vi "UHR-Fleezers Control (host) - 11.9b.vi"() -> ()   [LabVIEW 2014] (continued)
                n2360 = call "Create new save file.vi"("Insert"="video_frame_" ("string"), "Ext"=".bmp" ("string"), "Index In"="Image Index") -> ("Path Out"=w3445:path, "Index Out"=w3450:dbl)
                n2361 = Increment(x=w3450) -> (x+1=w3444:dbl)
                n2362 = local write "Image Index"(w3444) -> ()
                n2363 = call <vilib>:"Write BMP File.vi"("image data"=w3449, "path to BMP file"=w3445) -> ()  [unwired: 1 in, 9 out]
              }
            }
            n2364 = case shown="True" "Target" {
              tunnel: w3363 -> [w3389 w3393]
              tunnel: [w3389 w3391] -> w3362
              frame False {
              }
              frame True {
                n2365 = local read "Target coordinates"() -> (w3390:cluster{"X1":dbl, "Y1":dbl, "X2":dbl, "Y2":dbl})
                n2366 = call "IMAQ Overlay Oval"("Color"=u32 16711680, "Bounding Rectangle"=w3390, "Image"=w3393) -> ("Image Out"=w3391:T2)  [unwired: 7 in, 1 out]
              }
            }
            "Primary Video Display" <- w3362
          }
        }
        n2367 = node-c288(w3324) -> ()  [unwired: 1 out]
      }
      n2368 = node-c288(w3308) -> ()  [unwired: 1 out]
      n2369 = call "DMR_CloseDevice2.vi"("driver handle IN"=w3313) -> ()  [unwired: 1 in, 4 out]
    }
    frame #4 {
      n2370 = call "DMR_Close.vi"() -> ()  [unwired: 1 out]
    }
  }
  n2371 = local write "Offset (nm)"(0.0 ("Offset (nm)")) -> ()
  n2372 = local write "Bead Mean (nm)"(0.0 ("Bead Mean (nm)")) -> ()
  n2373 = local write "Total Volume\nFlowed P1 (uL)"(w17) -> ()
  n2374 = local write "Total Volume\nFlowed Samp (uL)"(w17) -> ()
  n2375 = local write "Total Volume\nFlowed P3 (uL)"(w17) -> ()
  n2376 = node-c288(i64 1 ("Period"), 1 ("Processor")) -> (w196:T21)  [unwired: 2 out]
  n2377 = timed-loop "Acquire Data" {
    tunnel: w23 -> [w3758]
    tunnel: w72 -> [w3757]
    tunnel: [w3787] -> w289
    tunnel: [w3782] -> w287
    timing: w196 -> [_]
    timing-out: [_] -> w195
    tunnel: w91 -> [w3597]
    stop <- "Stop All" stop-if-true
    w3515 = "Initialize"
    w3584 = "NI_ChannelName" ("name")
    # "I think that the conversion\nfrom 'wiggle amp' to nm\nis 0.277 nm/input. So, 1000\nfor an input is 277 nm."
    n2378 = node-c288() -> ()  [unwired: 2 out]
    n2379 = First Call?() -> (First Call?: T/F=w3550:bool)
    n2380 = Or(x="Reset", y=w3550) -> (x .or. y?=w3551:bool)
    n2381 = local read "Flushing P1"() -> (w3470:bool)
    n2382 = case "Reset data stream" shown="True" w3551 {
      tunnel: w3758 -> [w4825 w4833]
      tunnel: w3757 -> [w4824 w4832]
      tunnel: [w4825 w4827] -> w3463
      tunnel: [w4824 w4826] -> w3753
      frame False {
      }
      frame True {
        w4830 = TRUE ("AI to FIFO")
        n2383 = local write "Overflow (data lost)"(FALSE ("Overflow (data lost)")) -> ()
        n2384 = call "reset FPGA DMA.vi"("error in"=w4832, "FPGA VI Reference In"=w4833) -> ("error out"=w4828:errorcluster, "FPGA VI Reference Out"=w4829:T19)
        n2385 = xnode "Read/Write Control"("FPGA VI Reference In"=w4829, "error in"=w4828, "AI to FIFO"=w4830, "APD to FIFO"=w4830) -> ("FPGA VI Reference Out"=w4827:T19, "error out"=w4826:errorcluster)
      }
    }
    n2386 = case shown="True" w3470 {
      frame False {
      }
      frame True {
        n2387 = local read "Flush rate (uL/m) P1"() -> (w3860:dbl)
        n2388 = local read "HP1 Flush Time (s)"() -> (w3866:dbl)
        n2389 = local read "DMA Update Period (s)"() -> (w3853:dbl)
        n2390 = Divide(x=w3860, y=60.0) -> (x/y=w3852:dbl)
        n2391 = feedback #4(0.0) -> (w3855:dbl)
        n2392 = Divide(x=w3866, y=w3853) -> (x/y=w3858:dbl)
        n2393 = feedback #5(0) -> (w3864:i32)
        n2394 = Increment(x=w3864) -> (x+1=w3857:i32)
        n2395 = Multiply(x=w3853, y=w3852) -> (x*y=w3851:dbl)
        n2396 = Greater?(x=w3857, y=w3858) -> (0:w3863:bool)
        n2397 = Compound Arithmetic op=MULTIPLY(w3853, w3857, w3852) -> (→"P1 Flush Volume (uL)":dbl)
        n2398 = Divide(x=w3857, y=w3858) -> (x/y=→"P1 Flushing Bar":dbl)
        n2399 = Add(x=w3851, y=w3855) -> (x+y=w3854:dbl)
        "Total Volume\nFlowed P1 (uL)" <- w3854
        n2400 = feedback-in #4(w3854) -> ()
        n2401 = case shown="True" w3863 {
          tunnel: w3857 -> [w3867 _]
          tunnel: [w3867 0] -> w3862
          frame False {
          }
          frame True {
            w3868 = FALSE ("Flushing P1")
            n2402 = local write "Inject Pump 1"(w3868) -> ()
            n2403 = local write "Flushing P1"(w3868) -> ()
            n2404 = property on="Clear Volume P1" class="Bool (strict)"("Val(Sgnl)"=TRUE ("Value (Signaling)")) -> ()  [unwired: 2 in, 2 out]
          }
        }
        n2405 = feedback-in #5(w3862) -> ()
      }
    }
    n2406 = Or(x="Start AOD Scan", y="Trap Raster Scan") -> (x .or. y?=w3705:bool)
    n2407 = case "Start AOM raster scan" shown="True" w3705 {
      tunnel: w3463 -> [w4675 w4685]
      tunnel: w3753 -> [w4674 w4684]
      tunnel: [w4675 w4678] -> w3455
      tunnel: [w4674 w4677] -> w3752
      frame False {
      }
      frame True {
        n2408 = case shown="True" "Restart DMA? (AOD)" {
          tunnel: [w4723 w4725] -> w4679
          tunnel: [w4722 w4724] -> w4680
          tunnel: w4685 -> [w4723 w4727]
          tunnel: w4684 -> [w4722 w4726]
          frame False {
          }
          frame True {
            n2409 = local write "Overflow (data lost)"(FALSE ("Overflow (data lost)")) -> ()
            n2410 = call "reset FPGA DMA.vi"("error in"=w4726, "FPGA VI Reference In"=w4727) -> ("error out"=w4724:errorcluster, "FPGA VI Reference Out"=w4725:T19)
          }
        }
        n2411 = local write "Trap Raster Scan"(FALSE ("Trap Raster Scan")) -> ()
        n2412 = case shown="False" "Move MCL Also?" {
          tunnel: w4680 -> [w4689 w4717]
          tunnel: w4679 -> [w4690 w4718]
          tunnel: [w4688 w4721] -> w4678
          tunnel: [w4687 w4720] -> w4677
          frame False {
            w4686 = TRUE ("AI to FIFO")
            n2413 = xnode "Read/Write Control"("FPGA VI Reference In"=w4690, "error in"=w4689, "AI to FIFO"=w4686, "APD to FIFO"=w4686, "Start scan"=w4686) -> ("FPGA VI Reference Out"=w4688:T19, "error out"=w4687:errorcluster)
          }
          frame True {
            w4714 = FALSE ("1D or 2D Scan?")
            w4719 = TRUE ("AI to FIFO")
            # "Count for MCL loop"
            # "N total cycles"
            # "N steps"
            # "V_int"
            n2414 = local read "Scan Range (nm)"() -> (w4696:dbl)
            n2415 = local read "Number of F/B Scans (AOD)"() -> (w4713:u16)
            n2416 = Sign(1:w4696) -> (0:w4695:dbl)
            n2417 = Compound Arithmetic op=MULTIPLY(w4696, "MCL Step Position Ratio", "MCL/AOM Scale Tweak") -> (w4700:dbl)
            n2418 = Negate(x=w4695) -> (-x=w4692:dbl)
            n2419 = Multiply(x=w4692, y="MCL Step Increment (V_int)") -> (x*y=w4694:dbl)
            n2420 = Divide(x=w4700, y="MCL X Cal (nm/V)") -> (x/y=w4706:dbl)
            n2421 = Multiply(x=32767.0 ("y"), y=w4706) -> (x*y=w4712:dbl)
            n2422 = local read "Total Counts (ticks)"() -> (w4697:u32)
            n2423 = local read "Cycles/step (AOD)"() -> (w4708:u64)
            n2424 = local read "Scan steps (AOD)"() -> (w4709:u64)
            n2425 = Divide(x=w4712, y=10.0) -> (x/y=w4705:dbl)
            n2426 = Divide(x=w4705, y="MCL Step Increment (V_int)") -> (x/y=w4703:dbl)
            n2427 = Absolute Value(x=w4703) -> (abs(x)=w4691:dbl)
            n2428 = Compound Arithmetic op=MULTIPLY(w4709, w4708, w4697) -> (w4704:u64)
            n2429 = local write "wait to reset values"(w4719) -> ()
            n2430 = local write "MCL Scanning"(w4719) -> ()
            n2431 = Divide(x=w4704, y=w4691) -> (x/y=w4701:dbl)
            "MCL Count" <- w4701
            n2432 = xnode "Read/Write Control"("FPGA VI Reference In"=w4718, "error in"=w4717, "Scan steps (MCL)"=w4691, "Number of scans (MCL)"=w4713, "Cycles per step (MCL)"=u64 1, "Scan freq.  increment (MCL)"=w4694, "1D or 2D Scan?"=w4714, "MCL Scan Axis"=w4714, "Cont. Scan (MCL)"=w4714, "MCL count"=w4701) -> ("FPGA VI Reference Out"=w4716:T19, "error out"=w4715:errorcluster)
            n2433 = xnode "Read/Write Control"("FPGA VI Reference In"=w4716, "error in"=w4715, "AI to FIFO"=w4719, "APD to FIFO"=w4719, "Start scan"=w4719, "Start scan (MCL)"=w4719) -> ("FPGA VI Reference Out"=w4721:T19, "error out"=w4720:errorcluster)
          }
        }
        "Raster Scanning..." <- TRUE ("Scanning...")
      }
    }
    n2434 = local read "Flushing P3"() -> (w3471:bool)
    n2435 = case "Keep track of when Harvard Pump 3 is done flushing" shown="True" w3471 {
      frame False {
      }
      frame True {
        n2436 = local read "Flush rate (uL/m) P3"() -> (w3879:dbl)
        n2437 = local read "DMA Update Period (s)"() -> (w3873:dbl)
        n2438 = local read "HP3 Flush Time (s)"() -> (w3887:dbl)
        n2439 = Divide(x=w3879, y=60.0) -> (x/y=w3874:dbl)
        n2440 = feedback #6(0) -> (w3885:i32)
        n2441 = Increment(x=w3885) -> (x+1=w3880:i32)
        n2442 = Divide(x=w3887, y=w3873) -> (x/y=w3881:dbl)
        n2443 = Multiply(x=w3873, y=w3874) -> (x*y=w3872:dbl)
        n2444 = Greater?(x=w3880, y=w3881) -> (0:w3884:bool)
        n2445 = feedback #7(0.0) -> (w3875:dbl)
        n2446 = Compound Arithmetic op=MULTIPLY(w3873, w3880, w3874) -> (→"P3 Flush Volume (uL)":dbl)
        n2447 = case shown="True" w3884 {
          tunnel: w3880 -> [w3888 _]
          tunnel: [w3888 0] -> w3883
          frame False {
          }
          frame True {
            w3889 = FALSE ("Flushing P3")
            n2448 = local write "Inject Pump 3"(w3889) -> ()
            n2449 = local write "Flushing P3"(w3889) -> ()
            n2450 = property on="Clear Volume P3" class="Bool (strict)"("Val(Sgnl)"=TRUE ("Value (Signaling)")) -> ()  [unwired: 2 in, 2 out]
          }
        }
        n2451 = feedback-in #6(w3883) -> ()
        n2452 = Divide(x=w3880, y=w3881) -> (x/y=→"P3 Flushing Bar":dbl)
        n2453 = Add(x=w3872, y=w3875) -> (x+y=w3876:dbl)
        "Total Volume\nFlowed P3 (uL)" <- w3876
        n2454 = feedback-in #7(w3876) -> ()
      }
    }
    n2455 = And(x="Save scans", y=w3705) -> (x .and. y?=w3751:bool)
    n2456 = local read "Flushing samp"() -> (w3464:bool)
    n2457 = case shown="True" w3464 {
      frame False {
      }
      frame True {
        n2458 = local read "DMA Update Period (s)"() -> (w3832:dbl)
        n2459 = local read "Flush rate (mL/m)"() -> (w3844:dbl)
        n2460 = local read "Samp Flush Time (s)"() -> (w3845:dbl)
        n2461 = Divide(x=w3844, y=60.0) -> (x/y=w3831:dbl)
        n2462 = feedback #8(0) -> (w3837:i32)
        n2463 = Increment(x=w3837) -> (x+1=w3836:i32)
        n2464 = Divide(x=w3845, y=w3832) -> (x/y=w3841:dbl)
        n2465 = Multiply(x=w3832, y=w3831) -> (x*y=w3830:dbl)
        n2466 = Greater?(x=w3836, y=w3841) -> (0:w3840:bool)
        n2467 = feedback #9(0.0) -> (w3833:dbl)
        n2468 = Compound Arithmetic op=MULTIPLY(w3832, w3836, w3831) -> (→"Samp Volume (uL)":dbl)
        n2469 = Divide(x=w3836, y=w3841) -> (x/y=→"Samp flush bar":dbl)
        n2470 = case shown="True" w3840 {
          tunnel: [w3846 0] -> w3839
          tunnel: w3836 -> [w3846 _]
          frame False {
          }
          frame True {
            w3849 = FALSE ("Flushing samp")
            n2471 = local write "Sample Channel\nFlow"(w3849) -> ()
            n2472 = local write "Flushing samp"(w3849) -> ()
            n2473 = property on="Clear Volume" class="Bool (strict)"("Val(Sgnl)"=TRUE) -> ()  [unwired: 2 in, 2 out]
          }
        }
        n2474 = feedback-in #8(w3839) -> ()
        n2475 = Add(x=w3830, y=w3833) -> (x+y=w3834:dbl)
        "Total Volume\nFlowed Samp (uL)" <- w3834
        n2476 = feedback-in #9(w3834) -> ()
      }
    }
    n2477 = Compound Arithmetic op=OR("Start MCL Scan", "Confocal\nImage", "Confocal\nLinescan") -> (w3703:bool)
    n2478 = And(x="Save Data (MCL)", y=w3703) -> (x .and. y?=w3750:bool)
    n2479 = case "Start MCL raster scan" shown="True" w3703 {
      tunnel: w3455 -> [w4292 w4308]
      tunnel: w3752 -> [w4291 w4307]
      tunnel: [w4292 w4303] -> w3462
      tunnel: [w4291 w4302] -> w3460
      tunnel: [FALSE w4301] -> w3736
      tunnel: "Start MCL Scan" -> [_ w4296]
      tunnel: "Confocal\nImage" -> [_ w4295]
      tunnel: "Confocal\nLinescan" -> [_ _]
      frame False {
      }
      frame True {
        w4301 = TRUE
        n2480 = case shown="True" "Restart DMA? (MCL)" {
          tunnel: [w4353 w4355] -> w4306
          tunnel: [w4352 w4354] -> w4305
          tunnel: w4308 -> [w4353 w4358]
          tunnel: w4307 -> [w4352 w4357]
          frame False {
          }
          frame True {
            n2481 = call "reset FPGA DMA.vi"("error in"=w4357, "FPGA VI Reference In"=w4358) -> ("error out"=w4354:errorcluster, "FPGA VI Reference Out"=w4355:T19)
            n2482 = local write "Overflow (data lost)"(FALSE ("Overflow (data lost)")) -> ()
          }
        }
        n2483 = case shown="False" w4296 {
          selector: w4296 -> [_ w4312]
          tunnel: w4295 -> [w4311 _]
          tunnel: [w4311 w4312] -> w4294
          frame False {
            n2484 = property on="2D or 1D Scan" class="Bool (strict)"("Val(Sgnl)"=w4311) -> ()  [unwired: 2 in, 2 out]
            n2485 = property on="Confocal\nImage" class="Bool (strict)"("Value"=FALSE ("Start Confocal Map")) -> ()  [unwired: 2 in, 2 out]
          }
          frame True {
          }
        }
        n2486 = local write "MCL Scanning"(w4301) -> ()
        n2487 = local read "AO1"() -> (w4298:dbl)
        n2488 = local read "AO2"() -> (w4297:dbl)
        n2489 = case shown="True" "Center Scan" {
          tunnel: w4306 -> [w4319 w4351]
          tunnel: w4305 -> [w4318 w4350]
          tunnel: [w4317 w4349] -> w4303
          tunnel: [w4316 w4348] -> w4302
          tunnel: [w4314 w4335] -> w4300
          tunnel: [w4313 w4334] -> w4299
          tunnel: w4298 -> [w4314 w4340]
          tunnel: w4297 -> [w4313 w4343]
          tunnel: w4294 -> [_ _]
          frame False {
            w4315 = TRUE ("AI to FIFO")
            n2490 = xnode "Read/Write Control"("FPGA VI Reference In"=w4319, "error in"=w4318, "AI to FIFO"=w4315, "APD to FIFO"=w4315, "Start scan (MCL)"=w4315) -> ("FPGA VI Reference Out"=w4317:T19, "error out"=w4316:errorcluster)
          }
          frame True {
            w4347 = TRUE ("AI to FIFO")
            n2491 = local read "Scan steps (MCL)"() -> (w4326:u64)
            n2492 = local read "Scan lines (y)"() -> (w4322:u64)
            n2493 = local read "Fast Scan Dir"() -> (w4333:bool)
            n2494 = local read "Actual MCL Inc (V)"() -> (w4323:dbl)
            n2495 = Decrement(x=w4322) -> (x-1=w4321:u64)
            n2496 = Decrement(x=w4326) -> (x-1=w4325:u64)
            n2497 = Multiply(x=w4323, y=w4321) -> (x*y=w4320:dbl)
            n2498 = Divide(x=w4320, y=2.0) -> (x/y=w4330:dbl)
            n2499 = Multiply(x=w4323, y=w4325) -> (x*y=w4324:dbl)
            n2500 = Divide(x=w4324, y=2.0) -> (x/y=w4329:dbl)
            n2501 = Select(t=w4329, s=w4333, f=w4330) -> (s? t:f=w4328:dbl)
            n2502 = Select(t=w4330, s=w4333, f=w4329) -> (s? t:f=w4332:dbl)
            n2503 = Subtract(x=w4340, y=w4332) -> (x-y=w4331:dbl)
            n2504 = Subtract(x=w4343, y=w4328) -> (x-y=w4327:dbl)
            n2505 = local read "2D or 1D Scan"() -> (w4345:bool)
            n2506 = Not(x=w4333) -> (.not. x?=w4339:bool)
            n2507 = Not(x=w4345) -> (.not. x?=w4341:bool)
            n2508 = And(x=w4333, y=w4341) -> (x .and. y?=w4342:bool)
            n2509 = And(x=w4341, y=w4339) -> (x .and. y?=w4344:bool)
            n2510 = Select(t=w4343, s=w4344, f=w4327) -> (s? t:f=w4334:dbl)
            n2511 = Select(t=w4340, s=w4342, f=w4331) -> (s? t:f=w4335:dbl)
            n2512 = call "Volt to I16.vi"("Voltage In"=w4335) -> ("I16 Voltage Out"=w4338:i16)
            n2513 = call "Volt to I16.vi"("Voltage In"=w4334) -> ("I16 Voltage Out"=w4337:i16)
            n2514 = xnode "Read/Write Control"("FPGA VI Reference In"=w4351, "error in"=w4350, "AI to FIFO"=w4347, "APD to FIFO"=w4347, "Start scan (MCL)"=w4347, "AO1"=w4338, "AO2"=w4337) -> ("FPGA VI Reference Out"=w4349:T19, "error out"=w4348:errorcluster)
          }
        }
        "Initial Y" <- w4300
        "Initial X" <- w4299
        n2515 = local write "Tab Control 6"(T3."Imaging" ("Tab Control 6")) -> ()
        "wait to reset values" <- w4301
      }
    }
    n2516 = case shown="True" "Wiggle" {
      selector: "Wiggle" -> [w3803 _]
      tunnel: w3462 -> [w3805 w3818]
      tunnel: [w3802 w3821] -> w3461
      tunnel: w3460 -> [w3804 w3816]
      tunnel: [w3801 w3820] -> w3459
      frame False {
        n2517 = xnode "Read/Write Control"("FPGA VI Reference In"=w3805, "error in"=w3804, "Wiggle trap 1"=w3803) -> ("FPGA VI Reference Out"=w3802:T19, "error out"=w3801:errorcluster)
      }
      frame True {
        w3810 = FALSE ("Abort wiggle")
        w3814 = TRUE
        n2518 = local read "Restart DMA? (AOD)"() -> (w3819:bool)
        n2519 = case shown="True" w3819 {
          tunnel: w3818 -> [w3823 w3828]
          tunnel: [w3823 w3827] -> w3817
          tunnel: w3816 -> [w3822 w3826]
          tunnel: [w3822 w3825] -> w3815
          frame False {
          }
          frame True {
            n2520 = local write "Overflow (data lost)"(FALSE) -> ()
            n2521 = call "reset FPGA DMA.vi"("error in"=w3826, "FPGA VI Reference In"=w3828) -> ("error out"=w3825:errorcluster, "FPGA VI Reference Out"=w3827:T19)
          }
        }
        n2522 = local write "Wiggle"(FALSE) -> ()
        n2523 = xnode "Read/Write Control"("FPGA VI Reference In"=w3817, "error in"=w3815, "AI to FIFO"=w3814, "APD to FIFO"=w3814, "Wiggle trap 1"="Wiggle T1", "Wiggle freq 1 (Hz)"="Wiggle freq 1 (Hz)", "Wiggle amp 1"="Wiggle amp 1 (units?)", "Abort wiggle 1"=w3810, "Wiggle trap 2"="Wiggle T2", "Abort wiggle 2"=w3810, "Wiggle freq 2 (Hz)"="Wig Freq 2 (Hz)", "Wiggle amp 2"="Wig amp 2") -> ("FPGA VI Reference Out"=w3821:T19, "error out"=w3820:errorcluster)
      }
    }
    n2524 = local read "Trap Pos Elements/DMA read"() -> (w3593:u32)
    n2525 = local read "Trap AI Elements/DMA read"() -> (w3666:u32)
    n2526 = local read "APD Elements/DMA read"() -> (w3632:u32)
    n2527 = xnode "Get APD Data"("FPGA VI Reference In"=w3461, "error in"=w3459, "Number of Elements"=w3632, "Timeout (ms)"=-1) -> ("Data"=w3631:u32[], "Elements Remaining"=→"APD FIFO Elements Remaining":u32)  [unwired: 2 out]
    n2528 = xnode "Invoke Method"("FPGA VI Reference In"=w3461, "error in"=w3459, "Number of Elements"=w3593, "Timeout (ms)"=-1) -> ("Data"=w3557:u16[], "Elements Remaining"=→"Trap Pos FIFO El Remaining":u32)  [unwired: 2 out]
    n2529 = xnode "Get Trap Data"("FPGA VI Reference In"=w3461, "error in"=w3459, "Number of Elements"=w3666, "Timeout (ms)"=-1 ("Timeout")) -> ("FPGA VI Reference Out"=w3492:T19, "error out"=w3491:errorcluster, "Data"=w3558:i16[], "Elements Remaining"=w3795:u32)
    "FIFO El. Rem." <- w3795
    n2530 = local read "Trap AI FIFO Depth"() -> (w3797:u32)
    n2531 = Subtract(x=w3797, y=w3666) -> (x-y=w3796:u32)
    n2532 = Decimate 1D Array(w3557) -> (w3554:u16[], w3556:u16[], w3555:u16[])
    n2533 = Divide(x=w3795, y=w3796) -> (x/y=w3794:dbl)
    "Buffer Status" <- w3794
    n2534 = To Unsigned Long Integer(number=w3554) -> (unsigned 32bit integer=w3553:u32[])
    n2535 = Join Numbers(hi=w3556, lo=w3555) -> ((hi.lo)=w3552:u32[])
    n2536 = Equal?(x=w3794, y=1.0) -> (x = y?=w3792:bool)
    n2537 = Join Numbers(hi=w3553, lo=w3552) -> ((hi.lo)=w3546:u64[])
    n2538 = call "IR AOM word to freq - vec.vi"("Frequency Word In (double vec)"=w3546) -> ("Frequency Out"=w3592:dbl[])
    n2539 = case "Alert buffer overflow" shown="True" w3792 {
      frame False {
      }
      frame True {
        n2540 = call <vilib>:"Beep.vi"() -> ()  [unwired: 3 in, 9 out]
        "Overflow (data lost)" <- TRUE ("Overflow (data lost)")
      }
    }
    n2541 = Decimate 1D Array(w3592) -> (w3591:dbl[], w3590:dbl[])
    n2542 = Build Array(w3591, w3590) -> (w3589:dbl[][])
    n2543 = local read "Trap Sets"() -> (w3665:u32)
    n2544 = case "Deinterlace trap data, average down PSD" shown="2" w3665 {
      tunnel: w3558 -> [w4388 w4453]
      tunnel: [w4385 w4450] -> w3658
      tunnel: [w4388 w4452] -> w3549
      tunnel: "Detector Type" -> [w4387 w4448]
      tunnel: [w4386 w4451] -> w3657
      tunnel: [w4384 w4449] -> w3769
      frame 1, Default {
        n2545 = Divide(x=w4388, y=3276.7) -> (x/y=w4389:dbl[])
        n2546 = Decimate 1D Array(w4389) -> (w4398:dbl[], w4397:dbl[], w4396:dbl[], w4395:dbl[], w4394:dbl[], w4393:dbl[], w4392:dbl[], w4391:dbl[])
        n2547 = case shown="\"IR-QPD + PSD + FB-QPD position\"" w4387 {
          tunnel: w4398 -> [w4422 w4447]
          tunnel: w4397 -> [w4421 w4446]
          tunnel: w4396 -> [w4406 w4424]
          tunnel: w4395 -> [w4407 w4434]
          tunnel: w4394 -> [w4420 w4445]
          tunnel: w4393 -> [w4419 w4444]
          tunnel: w4392 -> [w4403 w4425]
          tunnel: w4391 -> [w4402 w4423]
          tunnel: [w4401 w4431] -> w4386
          tunnel: [w4400 w4430] -> w4385
          tunnel: [w4399 w4429] -> w4384
          frame "IR-QPD + PSD + FB-QPD", Default {
            w4399 = 0  # Channel pattern
            n2548 = Divide(x=w4422, y=w4407) -> (x/y=w4409:dbl[])
            n2549 = Divide(x=w4421, y=w4407) -> (x/y=w4408:dbl[])
            n2550 = Divide(x=w4420, y=w4403) -> (x/y=w4405:dbl[])
            n2551 = Divide(x=w4419, y=w4402) -> (x/y=w4404:dbl[])
            n2552 = Build Array(w4409, w4408, w4407, w4406, w4405, w4404, w4403, w4402) -> (w4400:dbl[][])
            n2553 = Bundle("T1 Y", "T1 X", "T1 Sum", "FB Sum", "PSD Y", "PSD X", "PSD Y Sum", "PSD X Sum") -> (w4418:T41)  [unwired: 1 out]
            n2554 = Cluster To Array(cluster=w4418) -> (array=w4401:string[])
          }
          frame "IR-QPD + PSD + FB-QPD position" {
            w4429 = 3  # Channel pattern
            n2555 = Negate(x=w4425) -> (-x=w4426:dbl[])
            n2556 = Divide(x=w4447, y=w4434) -> (x/y=w4436:dbl[])
            n2557 = Divide(x=w4446, y=w4434) -> (x/y=w4435:dbl[])
            n2558 = Divide(x=w4445, y=w4425) -> (x/y=w4433:dbl[])
            n2559 = Divide(x=w4444, y=w4426) -> (x/y=w4432:dbl[])
            n2560 = Build Array(w4436, w4435, w4434, w4423, w4424, w4433, w4432, w4425) -> (w4430:dbl[][])
            n2561 = Bundle("T1 Y", "T1 X", "T1 Sum", "FB X", "FB Sum", "PSD Y", "PSD X", "PSD Y Sum") -> (w4443:T41)  [unwired: 1 out]
            n2562 = Cluster To Array(cluster=w4443) -> (array=w4431:string[])
          }
        }
      }
      frame 2 {
        n2563 = case shown="\"IR-QPD + PSD + FB-QPD\", Default" w4448 {
          tunnel: w4453 -> [w4515 w4582 w4653]
          tunnel: [w4454 w4573 w4584] -> w4452
          tunnel: [w4481 w4564 w4631] -> w4451
          tunnel: [w4480 w4527 w4598] -> w4450
          tunnel: [w4474 w4562 w4629] -> w4449
          frame "IR-QPD + PSD + FB-QPD", Default {
            w4474 = 1  # Channel pattern
            # "time average x2 the 4th signal and the 4 psd signals (detection laser)"
            # "deinterlace 3 signals from qpd"
            n2564 = Decimate 1D Array(w4515) -> (w4514:i16[], w4513:i16[], w4479:i16[], w4512:i16[], w4502:i16[], w4500:i16[], w4499:i16[], w4497:i16[])
            n2565 = Decimate 1D Array(w4479) -> (w4478:i16[], w4477:i16[])
            n2566 = Decimate 1D Array(w4514) -> (w4511:i16[], w4483:i16[])
            n2567 = Decimate 1D Array(w4513) -> (w4510:i16[], w4508:i16[])
            n2568 = Decimate 1D Array(w4512) -> (w4509:i16[], w4507:i16[])
            n2569 = call "downsample 1D array - double.vi"("Ave N"=2.0, "Array In"=w4502) -> ("Array Out"=w4501:dbl[])  [unwired: 1 out]
            n2570 = call "downsample 1D array - double.vi"("Ave N"=2.0, "Array In"=w4500) -> ("Array Out"=w4482:dbl[])  [unwired: 1 out]
            n2571 = call "downsample 1D array - double.vi"("Ave N"=2.0, "Array In"=w4499) -> ("Array Out"=w4498:dbl[])  [unwired: 1 out]
            n2572 = call "downsample 1D array - double.vi"("Ave N"=2.0, "Array In"=w4497) -> ("Array Out"=w4496:dbl[])  [unwired: 1 out]
            n2573 = Interleave 1D Arrays(w4511, w4510, w4509, w4483, w4508, w4507, w4478, w4477, w4501, w4482, w4498, w4496) -> (w4495:dbl[])
            n2574 = Divide(x=w4495, y=3276.7) -> (x/y=w4494:dbl[])
            n2575 = Decimate 1D Array(w4494) -> (w4493:dbl[], w4492:dbl[], w4491:dbl[], w4490:dbl[], w4489:dbl[], w4488:dbl[], w4476:dbl[], w4475:dbl[], w4487:dbl[], w4486:dbl[], w4485:dbl[], w4484:dbl[])
            n2576 = Divide(x=w4493, y=w4491) -> (x/y=w4461:dbl[])
            n2577 = Divide(x=w4492, y=w4491) -> (x/y=w4460:dbl[])
            n2578 = Divide(x=w4490, y=w4488) -> (x/y=w4459:dbl[])
            n2579 = Divide(x=w4489, y=w4488) -> (x/y=w4458:dbl[])
            n2580 = Divide(x=w4487, y=w4485) -> (x/y=w4457:dbl[])
            n2581 = Divide(x=w4486, y=w4484) -> (x/y=w4456:dbl[])
            n2582 = Build Array(w4461, w4460, w4491, w4459, w4458, w4488, w4476, w4475, w4457, w4456, w4485, w4484) -> (w4480:dbl[][])
            n2583 = Bundle("T1 Y", "T1 X", "T1 Sum", "T2 Y", "T2 X", "T2 Sum", "T1 FB Sum", "T2 FB Sum", "PSD Y", "PSD X", "PSD Y Sum", "PSD X Sum") -> (w4462:T42)  [unwired: 1 out]
            n2584 = To Word Integer(number=w4495) -> (16bit integer=w4454:i16[])
            n2585 = Cluster To Array(cluster=w4462) -> (array=w4481:string[])
          }
          frame "IR-QPD + PSD + FB-QPD X position" {
            w4562 = 2  # Channel pattern
            # "time average x2 the 3 psd signals (detection laser)"
            # "deinterlace 3 signals from qpds"
            n2586 = Decimate 1D Array(w4582) -> (w4581:i16[], w4580:i16[], w4563:i16[], w4579:i16[], w4525:i16[], w4522:i16[], w4519:i16[], w4550:i16[])
            n2587 = Decimate 1D Array(w4563) -> (w4548:i16[], w4546:i16[])
            n2588 = Decimate 1D Array(w4581) -> (w4578:i16[], w4565:i16[])
            n2589 = Decimate 1D Array(w4580) -> (w4577:i16[], w4575:i16[])
            n2590 = Decimate 1D Array(w4579) -> (w4576:i16[], w4574:i16[])
            n2591 = Decimate 1D Array(w4550) -> (w4549:i16[], w4547:i16[])
            n2592 = call "downsample 1D array - I16.vi"("Ave N"=2.0, "Array In"=w4525) -> ("Array Out"=w4523:i16[])  [unwired: 1 in]
            n2593 = call "downsample 1D array - I16.vi"("Ave N"=2.0, "Array In"=w4519) -> ("Array Out"=w4517:i16[])  [unwired: 1 in]
            n2594 = call "downsample 1D array - I16.vi"("Ave N"=2.0, "Array In"=w4522) -> ("Array Out"=w4520:i16[])  [unwired: 1 in]
            n2595 = Interleave 1D Arrays(w4578, w4577, w4576, w4565, w4575, w4574, w4549, w4548, w4547, w4546, w4523, w4520, w4517) -> (w4573:i16[])
            n2596 = Divide(x=w4573, y=3276.7) -> (x/y=w4572:dbl[])
            n2597 = Decimate 1D Array(w4572) -> (w4571:dbl[], w4570:dbl[], w4569:dbl[], w4568:dbl[], w4567:dbl[], w4566:dbl[], w4538:dbl[], w4536:dbl[], w4535:dbl[], w4533:dbl[], w4532:dbl[], w4531:dbl[], w4528:dbl[])
            n2598 = Negate(x=w4528) -> (-x=w4526:dbl[])
            n2599 = Divide(x=w4532, y=w4528) -> (x/y=w4530:dbl[])
            n2600 = Divide(x=w4531, y=w4526) -> (x/y=w4529:dbl[])
            n2601 = Divide(x=w4571, y=w4569) -> (x/y=w4554:dbl[])
            n2602 = Divide(x=w4570, y=w4569) -> (x/y=w4553:dbl[])
            n2603 = Divide(x=w4568, y=w4566) -> (x/y=w4552:dbl[])
            n2604 = Divide(x=w4567, y=w4566) -> (x/y=w4551:dbl[])
            n2605 = Divide(x=w4538, y=w4536) -> (x/y=w4537:dbl[])
            n2606 = Divide(x=w4535, y=w4533) -> (x/y=w4534:dbl[])
            n2607 = Build Array(w4554, w4553, w4569, w4552, w4551, w4566, w4537, w4536, w4534, w4533, w4530, w4529, w4528) -> (w4527:dbl[][])
            n2608 = Bundle("T1 Y", "T1 X", "T1 Sum", "T2 Y", "T2 X", "T2 Sum", "T1 FB X", "T1 FB Sum", "T2 FB X", "T2 FB Sum", "PSD Y", "PSD X", "PSD Y Sum") -> (w4555:T43)  [unwired: 1 out]
            n2609 = Cluster To Array(cluster=w4555) -> (array=w4564:string[])
          }
          frame "IR-QPD + PSD + FB-QPD XY positions" {
            w4629 = 4  # Channel pattern
            # "time average x2 the 3 psd signals (detection laser)"
            # "deinterlace 3 signals from qpds"
            n2610 = Decimate 1D Array(w4653) -> (w4652:i16[], w4651:i16[], w4630:i16[], w4650:i16[], w4596:i16[], w4642:i16[], w4641:i16[], w4618:i16[])
            n2611 = Decimate 1D Array "Feedback Sum"(w4630) -> (w4614:i16[], w4612:i16[])
            n2612 = Decimate 1D Array "QPD Y"(w4652) -> (w4649:i16[], w4632:i16[])
            n2613 = Decimate 1D Array "QPD X"(w4651) -> (w4648:i16[], w4646:i16[])
            n2614 = Decimate 1D Array "Feedback Y"(w4596) -> (w4595:i16[], w4594:i16[])
            n2615 = Decimate 1D Array "QPD Sum"(w4650) -> (w4647:i16[], w4645:i16[])
            n2616 = Decimate 1D Array "Feedback X"(w4618) -> (w4615:i16[], w4613:i16[])
            n2617 = call "downsample 1D array - double.vi"("Ave N"=2.0, "Array In"=w4642) -> ("Array Out"=w4617:dbl[])  [unwired: 1 out]
            n2618 = call "downsample 1D array - double.vi"("Ave N"=2.0, "Array In"=w4641) -> ("Array Out"=w4616:dbl[])  [unwired: 1 out]
            n2619 = Interleave 1D Arrays(w4649, w4648, w4647, w4632, w4646, w4645, w4595, w4615, w4614, w4594, w4613, w4612, w4617, w4616) -> (w4640:dbl[])
            n2620 = Divide(x=w4640, y=3276.7) -> (x/y=w4639:dbl[])
            n2621 = Decimate 1D Array(w4639) -> (w4638:dbl[], w4637:dbl[], w4636:dbl[], w4635:dbl[], w4634:dbl[], w4633:dbl[], w4591:dbl[], w4605:dbl[], w4589:dbl[], w4590:dbl[], w4603:dbl[], w4587:dbl[], w4601:dbl[], w4599:dbl[])
            n2622 = Negate(x=w4599) -> (-x=w4597:dbl[])
            n2623 = Divide(x=w4601, y=w4597) -> (x/y=w4600:dbl[])
            n2624 = Divide(x=w4590, y=w4587) -> (x/y=w4586:dbl[])
            n2625 = Divide(x=w4591, y=w4589) -> (x/y=w4588:dbl[])
            n2626 = Divide(x=w4638, y=w4636) -> (x/y=w4622:dbl[])
            n2627 = Divide(x=w4637, y=w4636) -> (x/y=w4621:dbl[])
            n2628 = Divide(x=w4635, y=w4633) -> (x/y=w4620:dbl[])
            n2629 = Divide(x=w4634, y=w4633) -> (x/y=w4619:dbl[])
            n2630 = Divide(x=w4605, y=w4589) -> (x/y=w4604:dbl[])
            n2631 = Divide(x=w4603, y=w4587) -> (x/y=w4602:dbl[])
            n2632 = Build Array(w4622, w4621, w4636, w4620, w4619, w4633, w4588, w4604, w4589, w4586, w4602, w4587, w4600, w4599) -> (w4598:dbl[][])
            n2633 = Bundle("T1 Y", "T1 X", "T1 Sum", "T2 Y", "T2 X", "T2 Sum", "T1 FB Y", "T1 FB X", "T1 FB Sum", "T2 FB Y", "T2 FB X", "T2 FB Sum", "PSD X", "PSD Y Sum") -> (w4585:T44)  [unwired: 1 out]
            n2634 = To Word Integer(number=w4640) -> (16bit integer=w4584:i16[])
            n2635 = Cluster To Array(cluster=w4585) -> (array=w4631:string[])
          }
        }
      }
    }
    "AI labels" <- w3657
    n2636 = Decimate 1D Array(w3631) -> (w3655:u32[], w3599:u32[])
    n2637 = local read "DMA Update Period (s)"() -> (w3667:dbl)
    n2638 = Build Array(w3655, w3599) -> (w3733:u32[][])
    n2639 = local read "Data Period (s)"() -> (w3508:dbl)
    n2640 = local read "BD 1 Frequency 2 (MHz)"() -> (w3541:dbl)
    n2641 = local read "BD 1 Frequency 1 (MHz)"() -> (w3542:dbl)
    n2642 = Decimate 1D Array(w3549) -> (w3572:i16[], w3571:i16[], w3569:i16[], w3568:i16[])  [unwired: 9 out]
    n2643 = To Double Precision Float(number=w3733) -> (double precision float=w3734:dbl[][])
    n2644 = local read "APD Integration Time (s)"() -> (w3612:dbl)
    n2645 = Multiply(x=w3508, y="Trap Pos. Disp. Downsample") -> (x*y=w3506:dbl)
    n2646 = Divide(x=w3572, y=w3571) -> (x/y=w3573:dbl[])
    n2647 = Divide(x=w3569, y=w3568) -> (x/y=w3570:dbl[])
    n2648 = feedback #10(0.0) -> (w3586:dbl)
    n2649 = Add(x=w3667, y=w3586) -> (x+y=w3771:dbl)
    n2650 = feedback-in #10(w3771) -> ()
    n2651 = local read "AOM X Cal (nm/MHz)"() -> (w3539:dbl)
    n2652 = To Time Stamp(1:w3586) -> (0:w3585:timestamp)
    n2653 = Split 1D Array(array=w3573, index="N El. to Ave.") -> (second subarray=w3576:dbl[])  [unwired: 1 out]
    n2654 = Split 1D Array(array=w3570, index="N El. to Ave.") -> (second subarray=w3575:dbl[])  [unwired: 1 out]
    n2655 = Multiply(x=w3508, y="Trap Disp. Downsample") -> (x*y=w3587:dbl)
    "Display Period (s)" <- w3587
    n2656 = for "Trap AI" {
      tunnel: [w4383] -> w3765 mode=indexing
      tunnel: w3585 -> [w4373]
      tunnel: "Trap Disp. Downsample" -> [w4381]
      tunnel: w3658 -> [w4379] mode=indexing
      tunnel: w3508 -> [w4378]
      tunnel: w3657 -> [w4377] mode=indexing
      tunnel: w3584 -> [w4376]
      tunnel: [w4375] -> w3623 mode=indexing
      tunnel: w3587 -> [w4374]
      workers-P: _ -> [_]
      n2657 = Bundle By Name("Y"=w4379, "dt"=w4378) -> (w4380:waveform(dbl))  [unwired: 1 out]
      n2658 = Set Waveform Attribute(5:w4377, 6:w4376, 7:w4380) -> (3:w4375:waveform(dbl))  [unwired: 1 in, 2 out]
      n2659 = call "downsample 1D array - double.vi"("Ave N"=w4381, "Array In"=w4379) -> ("Array Out"=w4382:dbl[])  [unwired: 1 out]
      n2660 = Bundle By Name(cluster=w4375, "t0"=w4373, "Y"=w4382, "dt"=w4374) -> (w4383:waveform(dbl))
    }
    n2661 = Bundle("BD 1 Frequency 1 (MHz)"=w3542, "BD 1 Frequency 2 (MHz)"=w3541) -> (w3543:T45)  [unwired: 1 out]
    n2662 = call-poly <vilib>:"Mean.vi"("X"=w3575) -> ("mean"=w3563:dbl)  [unwired: 1 out]
    n2663 = call-poly <vilib>:"Mean.vi"("X"=w3576) -> ("mean"=w3564:dbl)  [unwired: 1 out]
    n2664 = Reciprocal(x=w3587) -> (1/x=→"Trap Disp. Freq. (Hz)":dbl)
    n2665 = Cluster To Array(cluster=w3543) -> (array=w3540:dbl[])
    n2666 = local read "Trap X AI1 (DMA)"() -> (w3574:T13)
    n2667 = local read "Data points/scans (MCL)"() -> (w3745:dbl)
    n2668 = To Fixed-Point(number=w3563) -> (fixed-point=w3561:fxp<+/-,16,1>)  [unwired: 1 in]
    n2669 = To Fixed-Point(number=w3564) -> (fixed-point=w3562:fxp<+/-,16,1>)  [unwired: 1 in]
    n2670 = Bundle("Trap 1 Pos.", "Trap 2 Pos.") -> (w3583:cluster{string, string})  [unwired: 1 out]
    n2671 = Bundle By Name(cluster=w3574, "Set 1"=w3562, "Set 2"=w3561) -> (→"Trap X AI1 (DMA)":T13)
    n2672 = Cluster To Array(cluster=w3583) -> (array=w3580:string[])
    n2673 = Bundle("APD 1", "APD 2") -> (w3764:cluster{string, string})  [unwired: 1 out]
    n2674 = Select(t=-1.0, s="Negate Y Axis", f=1.0) -> (s? t:f=w3525:dbl)
    n2675 = for "Trap Position" {
      tunnel: w3589 -> [w4017] mode=indexing
      tunnel: "Trap Pos. Disp. Downsample" -> [w4016]
      tunnel: w3506 -> [w4014]
      tunnel: w3585 -> [w4013]
      tunnel: w3584 -> [w4011]
      tunnel: w3580 -> [w4010] mode=indexing
      tunnel: [w4009] -> w3495 mode=indexing
      tunnel: w3540 -> [w4007] mode=indexing
      tunnel: w3539 -> [w4005]
      tunnel: w3525 -> [w4004]
      n2676 = call "downsample 1D array - double.vi"("Ave N"=w4016, "Array In"=w4017) -> ("Array Out"=w4015:dbl[])  [unwired: 1 out]
      n2677 = Subtract(x=w4015, y=w4007) -> (x-y=w4008:dbl[])
      n2678 = Multiply(x=w4005, y=w4008) -> (x*y=w4006:dbl[])
      n2679 = Multiply(x=w4004, y=w4006) -> (x*y=w4003:dbl[])
      n2680 = Bundle By Name("Y"=w4003, "dt"=w4014, "t0"=w4013) -> (w4012:waveform(dbl))  [unwired: 1 out]
      n2681 = Set Waveform Attribute(5:w4010, 6:w4011, 7:w4012) -> (3:w4009:waveform(dbl))  [unwired: 1 in, 2 out]
    }
    n2682 = Cluster To Array(cluster=w3764) -> (array=w3761:string[])
    n2683 = for "APD" {
      tunnel: w3734 -> [w4362] mode=indexing
      tunnel: w3612 -> [w4370]
      tunnel: [w4366] -> w3619 mode=indexing
      tunnel: "APD Disp. Scale" -> [w4367]
      tunnel: w3584 -> [w4365]
      tunnel: w3761 -> [w4364] mode=indexing
      tunnel: "APD Disp. Downsample" -> [w4360]
      tunnel: [w4363] -> w3760
      workers-P: _ -> [_]
      tunnel: w3585 -> [w4359]
      n2684 = call "integrate 1D array interval - double.vi"("Ave N"=w4360, "Array In"=w4362) -> ("Array Out"=w4361:dbl[])  [unwired: 1 out]
      n2685 = Multiply(x=w4370, y=w4360) -> (x*y=w4363:dbl)
      n2686 = Divide(x=w4361, y=w4367) -> (x/y=w4368:dbl[])
      n2687 = Bundle By Name("t0"=w4359, "Y"=w4368, "dt"=w4363) -> (w4369:waveform(dbl))  [unwired: 1 out]
      n2688 = Set Waveform Attribute(5:w4364, 6:w4365, 7:w4369) -> (3:w4366:waveform(dbl))  [unwired: 1 in, 2 out]
    }
    "APD Display Period (s)" <- w3760
    n2689 = Reciprocal(x=w3760) -> (1/x=→"APD Display Freq. (Hz)":dbl)
    n2690 = local read "Display Period (s)"() -> (w3643:dbl)
    n2691 = Increment(x=w3745) -> (x+1=w3746:dbl)
    n2692 = To Double Precision Float(number=w3655) -> (double precision float=w3654:dbl[])
    n2693 = Index Array(array=w3495, index=0) -> (element=w3499:waveform(dbl))
    n2694 = Index Array(array=w3495, index=1) -> (element=w3494:waveform(dbl))
    n2695 = feedback #11(w3746) -> (w3749:dbl)
    n2696 = Select(t=0, s=w3736, f=w3749) -> (s? t:f=w3742:dbl)
    n2697 = Array Size(array=w3654) -> (size(s)=w3748:i32)
    n2698 = Add(x=w3748, y=w3742) -> (x+y=w3743:dbl)
    n2699 = Unbundle By Name(w3499) -> ("Y"=w3500:dbl[])
    n2700 = feedback #12(w3655) -> (w3732:u32[])
    n2701 = Build Array (concatenate)(w3732, w3655) -> (w3729:u32[])
    n2702 = feedback #13(w3599) -> (w3618:u32[])
    n2703 = Divide(x="Bead Sep. Int. Time (s)", y=w3643) -> (x/y=w3535:dbl)
    n2704 = Build Array (concatenate)(w3618, w3599) -> (w3617:u32[])
    n2705 = Add(x=w3500, y="FB Trap Pos Offset") -> (x+y=w3498:dbl[])
    "T1 x pos data" <- w3498
    n2706 = Greater?(x=w3743, y=w3745) -> (0:w3744:bool)
    n2707 = feedback #14(w3498) -> (w3537:dbl[])
    n2708 = Build Array (concatenate)(w3498, w3537) -> (w3536:dbl[])
    n2709 = Bundle By Name(cluster=w3499, "Y"=w3498) -> (w3497:waveform(dbl))
    n2710 = Select(t=w3742, s=w3744, f=w3743) -> (s? t:f=w3741:dbl)
    n2711 = feedback-in #11(w3741) -> ()
    n2712 = Array Size(array=w3729) -> (size(s)=w3726:i32)
    n2713 = Array Size(array=w3655) -> (size(s)=w3728:i32)
    n2714 = local read "MCL Scanning"() -> (w3739:bool)
    n2715 = local read "APD Integration Time (s)"() -> (w3626:dbl)
    n2716 = Bundle(w3497, w3494) -> (w3493:cluster{waveform(dbl), waveform(dbl)})  [unwired: 1 out]
    n2717 = Build Array (concatenate)(w3619, w3765) -> (w3621:waveform(dbl)[])
    "All Signals" <- w3621
    n2718 = Split 1D Array(array=w3536, index=w3535) -> (first subarray=w3529:dbl[])  [unwired: 1 out]
    n2719 = feedback-in #14(w3529) -> ()
    n2720 = Multiply(x=w3728, y="APD Ave N") -> (x*y=w3727:dbl)
    n2721 = Greater?(x=w3726, y=w3727) -> (0:w3730:bool)
    n2722 = Not(x=w3744) -> (.not. x?=w3738:bool)
    n2723 = Cluster To Array(cluster=w3493) -> (array=w3469:waveform(dbl)[])
    "Trap Positions" <- w3469
    n2724 = To Double Precision Float(number=w3599) -> (double precision float=w3598:dbl[])
    n2725 = call-poly <vilib>:"Mean.vi"("X"=w3529) -> ("mean"=w3528:dbl)  [unwired: 1 out]
    "Mean T1 Position (nm)" <- w3528
    n2726 = Subtract(x=w3529, y=w3528) -> (x-y=w3534:dbl[])
    n2727 = Square(x=w3534) -> (x^2=w3533:dbl[])
    n2728 = And(x=w3738, y=w3739) -> (x .and. y?=w3740:bool)
    n2729 = call-poly <vilib>:"Mean.vi"("X"=w3533) -> ("mean"=w3532:dbl)  [unwired: 1 out]
    n2730 = case shown="True" w3730 {
      tunnel: w3729 -> [w4142 w4149]
      tunnel: [w4142 w4147] -> w3672
      tunnel: w3727 -> [_ w4144]
      tunnel: w3726 -> [_ w4148]
      tunnel: w3617 -> [w4141 w4146]
      tunnel: [w4141 w4143] -> w3614
      frame False {
      }
      frame True {
        n2731 = Subtract(x=w4148, y=w4144) -> (x-y=w4145:dbl)
        n2732 = Array Subset(array=w4149, index=w4145, length=w4144) -> (w4147:u32[])
        n2733 = Array Subset(array=w4146, index=w4145, length=w4144) -> (w4143:u32[])
      }
    }
    n2734 = feedback-in #12(w3672) -> ()
    n2735 = feedback-in #13(w3614) -> ()
    n2736 = Square Root(x=w3532) -> (sqrt(x)=w3531:dbl)
    n2737 = Or(x=w3740, y=w3736) -> (x .or. y?=w3737:bool)
    n2738 = Equal?(x="Tab Control 6", y=T35."High Res Display") -> (x = y?=w3661:bool)
    n2739 = Multiply(x="APD Disp. Scale", y=w3619) -> (x*y=w3628:waveform(dbl)[])
    n2740 = Multiply(x=10.0, y=w3531) -> (x*y=→"Trap 1 Position RMS (A)":dbl)
    n2741 = Multiply(x="APD Disp. Downsample", y=w3626) -> (x*y=w3624:dbl)
    n2742 = Divide(x=w3628, y=w3624) -> (x/y=w3596:waveform(dbl)[])
    n2743 = case "For displaying the high resolution display (no downsampling)" shown="True" w3661 {
      tunnel: w3623 -> [_ w4042]
      frame False {
      }
      frame True {
        n2744 = Index Array(array=w4042, index="High Res. Display") -> (element=w4043:waveform(dbl))
        n2745 = call <vilib>:"Std Deviation and Variance.vi"("X"=w4043) -> ("mean"=w4050:dbl, "standard deviation"=w4055:dbl)  [unwired: 1 in, 1 out]
        "Mean Intensity" <- w4050
        "Sigma" <- w4055
        n2746 = Subtract(x=w4043, y=w4050) -> (x-y=w4049:waveform(dbl))
        n2747 = Select(t=w4049, s="Subtract mean", f=w4043) -> (s? t:f=→"1 Channel":waveform(dbl))
        n2748 = Divide(x=w4055, y=w4050) -> (x/y=→"Sigma/Mean":dbl)
        n2749 = feedback #15(1) -> (w4044:i32)
        n2750 = Greater Or Equal?(x=w4044, y="Slow mean N ave.") -> (x >= y?=w4057:bool)
        n2751 = Increment(x=w4044) -> (x+1=w4059:i32)
        n2752 = Select(t=1, s=w4057, f=w4059) -> (s? t:f=w4046:i32)
        n2753 = feedback-in #15(w4046) -> ()
        n2754 = feedback #16() -> (w4047:waveform(dbl))  [unwired: 1 out]
        n2755 = case shown="Default" w4044 {
          tunnel: [w4062 w4065] -> w4048
          tunnel: w4047 -> [w4064 _]
          tunnel: w4043 -> [w4063 w4065]
          frame Default {
            n2756 = call-poly <vilib>:"Append Waveforms.vi"("waveform B"=w4063, "waveform A"=w4064) -> ("waveform out"=w4062:waveform(dbl))  [unwired: 1 in, 8 out]
          }
          frame 1 {
          }
        }
        n2757 = feedback-in #16(w4048) -> ()
        n2758 = case shown="True" w4057 {
          tunnel: w4048 -> [_ w4061]
          frame False {
          }
          frame True {
            n2759 = call-poly <vilib>:"Mean.vi"("X"=w4061) -> ("mean"=→"Slow mean":dbl)  [unwired: 1 out]
          }
        }
      }
    }
    n2760 = Index Array(array=w3596, index=0) -> (element=w3606:waveform(dbl))
    n2761 = Index Array(array=w3596, index=1) -> (element=w3604:waveform(dbl))
    n2762 = case "For computing FFTs for display" shown="True" "Compute FFT" {
      tunnel: w3623 -> [_ w4756]
      frame False {
      }
      frame True {
        n2763 = Build Array("FFT 1 Choice 1", "FFT 1 Choice 2", "FFT 2 Choice 1", "FFT 2 Choice 2") -> (w4749:u16[])
        n2764 = Array Size(array=w4756) -> (size(s)=w4755:i32)
        n2765 = feedback-in #17(w4749) -> ()
        n2766 = feedback #17(u16[] [100, 100, 100, 100]) -> (w4750:u16[])
        n2767 = feedback-in #18("# Spectra to Ave.") -> ()
        n2768 = feedback #18("# Spectra to Ave.") -> (w4747:dbl)
        n2769 = Not Equal?(x="# Spectra to Ave.", y=w4747) -> (x != y?=w4746:bool)
        n2770 = Not Equal?(x=w4749, y=w4750) -> (x != y?=w4748:bool)
        n2771 = feedback #19(1.0) -> (w4733:dbl)
        n2772 = Compound Arithmetic op=OR("Reset FFT", w4748, w4746) -> (w4731:bool)
        n2773 = Select(t=1.0, s=w4731, f=w4733) -> (s? t:f=w4735:dbl)
        n2774 = Greater?(x=w4735, y="# Spectra to Ave.") -> (0:w4754:bool)
        n2775 = Increment(x=w4735) -> (x+1=w4734:dbl)
        n2776 = feedback-in #19(w4734) -> ()
        n2777 = local read "DMA Update Period (s)"() -> (w4729:dbl)
        n2778 = Multiply(x="# Spectra to Ave.", y=w4729) -> (x*y=→"Ave. Time (s)":dbl)
        n2779 = Build Array(cluster{"f0":dbl, "df":dbl, "magnitude":dbl[]} {"f0"=0.0, "df"=0.0, "magnitude"=[]} ("PSD")) -> (w4738:cluster{"f0":dbl, "df":dbl, "magnitude":dbl[]}[])
        n2780 = Build Array(w4738, w4738, w4738, w4738) -> (w4740:T46)
        n2781 = feedback #20(w4740) -> (w4745:T46)
        n2782 = for {
          N: 4 -> [_]
          tunnel: w4749 -> [w4778] mode=indexing
          tunnel: w4756 -> [w4779]
          tunnel: w4755 -> [w4781]
          tunnel: w4731 -> [w4774]
          tunnel: w4754 -> [w4773]
          tunnel: "# Spectra to Ave." -> [w4772]
          tunnel: [w4771] -> w4744 mode=indexing
          tunnel: w4745 -> [w4776] mode=indexing
          tunnel: [w4775] -> w4732 mode=indexing
          tunnel: w4735 -> [w4770]
          n2783 = Less?(x=w4778, y=w4781) -> (x < y?=w4780:bool)
          n2784 = Index Array(array=w4779, index=w4778) -> (element=w4777:waveform(dbl))
          n2785 = case shown="True" w4780 {
            tunnel: w4777 -> [_ w4798]
            tunnel: w4776 -> [w4783 w4796]
            tunnel: [w4783 w4784] -> w4775
            tunnel: w4774 -> [_ w4795]
            tunnel: w4773 -> [_ w4788]
            tunnel: w4772 -> [_ w4787]
            tunnel: [cluster{"f0":dbl, "df":dbl, "magnitude":dbl[]} {"f0"=0.0, "df"=0.0, "magnitude"=[]} ("PSD") w4789] -> w4771
            tunnel: w4770 -> [_ w4786]
            frame False {
            }
            frame True {
              n2786 = call <vilib>:"Std Deviation and Variance.vi"("X"=w4798) -> ("mean"=w4799:dbl)  [unwired: 1 in, 2 out]
              n2787 = Subtract(x=w4798, y=w4799) -> (x-y=w4797:waveform(dbl))
              n2788 = xnode "Spectral Measurements"("Signals"=w4797) -> ("PSD"=w4791:cluster{"f0":dbl, "df":dbl, "magnitude":dbl[]})  [unwired: 1 in, 1 out]
              n2789 = case shown="False" w4795 {
                tunnel: w4796 -> [w4808 _]
                tunnel: [w4804 w4813] -> w4784
                tunnel: w4791 -> [w4807 w4814]
                tunnel: w4788 -> [w4806 _]
                frame False {
                  n2790 = Build Array (concatenate)(w4808, w4807) -> (w4805:cluster{"f0":dbl, "df":dbl, "magnitude":dbl[]}[])
                  n2791 = case shown="True" w4806 {
                    tunnel: w4805 -> [w4809 w4812]
                    tunnel: [w4809 w4810] -> w4804
                    frame False {
                    }
                    frame True {
                      n2792 = Delete From Array(array=w4812, index=0) -> (array with subset deleted=w4810:cluster{"f0":dbl, "df":dbl, "magnitude":dbl[]}[])  [unwired: 1 in, 1 out]
                    }
                  }
                }
                frame True {
                  n2793 = Build Array(w4814) -> (w4813:cluster{"f0":dbl, "df":dbl, "magnitude":dbl[]}[])
                }
              }
              n2794 = for {
                tunnel: w4784 -> [w4803] mode=indexing
                tunnel: [w4802] -> w4794 mode=indexing
                workers-P: _ -> [_]
                n2795 = Unbundle By Name(w4803) -> ("magnitude"=w4802:dbl[])
              }
              n2796 = Transpose 2D Array(2D array=w4794) -> (transposed array=w4793:dbl[][])
              n2797 = for {
                tunnel: w4793 -> [w4801] mode=indexing
                tunnel: [w4800] -> w4792 mode=indexing
                workers-P: _ -> [_]
                n2798 = Add Array Elements(numeric array=w4801) -> (sum=w4800:dbl)
              }
              n2799 = Select(t=w4787, s=w4788, f=w4786) -> (s? t:f=w4785:dbl)
              n2800 = Divide(x=w4792, y=w4785) -> (x/y=w4790:dbl[])
              n2801 = Bundle By Name(cluster=w4791, "magnitude"=w4790) -> (w4789:cluster{"f0":dbl, "df":dbl, "magnitude":dbl[]})
            }
          }
        }
        n2802 = case shown="True" w4731 {
          tunnel: w4732 -> [w4763 w4769]
          tunnel: [w4763 w4764] -> w4730
          frame False {
          }
          frame True {
            n2803 = Array Subset(array=w4769, index (row)=0 ("index"), length (row)=4 ("length"), index (col)=0 ("index"), length (col)=1 ("length")) -> (w4764:T46)
          }
        }
        n2804 = feedback-in #20(w4730) -> ()
        n2805 = Split 1D Array(array=w4744, index=2) -> (first subarray=→"FFT 1":cluster{"f0":dbl, "df":dbl, "magnitude":dbl[]}[], second subarray=→"FFT 2":cluster{"f0":dbl, "df":dbl, "magnitude":dbl[]}[])
      }
    }
    n2806 = case "For plotting results of scanning MCL" shown="True" w3737 {
      tunnel: w3736 -> [_ w4182]
      tunnel: w3654 -> [_ w4278]
      tunnel: w3745 -> [_ _]
      tunnel: w3623 -> [_ w4252]
      tunnel: w3598 -> [_ w4183]
      tunnel: w3597 -> [_ w4156]
      frame False {
      }
      frame True {
        w4163 = u32 0 items=["Horizontal", "Vertical", "Central", "1st Diagonal", "2nd Diagonal"] ("Type of Symmetry")
        w4191 = u32 0 items=["Horizontal", "Vertical", "Central", "1st Diagonal", "2nd Diagonal"] ("Type of Symmetry")
        w4194 = u32 0 items=["Horizontal", "Vertical", "Central", "1st Diagonal", "2nd Diagonal"] ("Type of Symmetry")
        w4223 = u32 0 items=["Horizontal", "Vertical", "Central", "1st Diagonal", "2nd Diagonal"] ("Type of Symmetry")
        n2807 = Index Array(array=w4252, index=10) -> (element=w4258:waveform(dbl))
        n2808 = Index Array(array=w4252, index=11) -> (element=w4255:waveform(dbl))
        n2809 = local read "Cycles/step (MCL)"() -> (w4208:u64)
        n2810 = Index Array(array=w4252, index="Channel") -> (element=w4254:waveform(dbl))
        n2811 = Unbundle(w4156) -> ("New Image"=w4155:T2, "New Image"=w4154:T2, "New Image"=w4153:T2, "New Image"=w4152:T2)
        n2812 = Unbundle By Name(w4258) -> ("Y"=w4210:dbl[])
        n2813 = Unbundle By Name(w4255) -> ("Y"=w4212:dbl[])
        n2814 = Unbundle By Name(w4254) -> ("Y"=w4217:dbl[])
        n2815 = call "downsample 1D array - double.vi"("Ave N"=w4208, "Array In"=w4210) -> ("Array Out"=w4209:dbl[])  [unwired: 1 out]
        n2816 = call "downsample 1D array - double.vi"("Ave N"=w4208, "Array In"=w4212) -> ("Array Out"=w4211:dbl[])  [unwired: 1 out]
        n2817 = call "downsample 1D array - double.vi"("Ave N"=w4208, "Array In"=w4217) -> ("Array Out"=w4216:dbl[])  [unwired: 1 out]
        n2818 = feedback #21(w4278) -> (w4279:dbl[])
        n2819 = Build Array (concatenate)(w4279, w4278) -> (w4260:dbl[])
        n2820 = feedback #22(w4183) -> (w4185:dbl[])
        n2821 = Build Array (concatenate)(w4185, w4183) -> (w4184:dbl[])
        n2822 = local read "Scan steps (MCL)"() -> (w4165:u64)
        n2823 = Select(t=w4278, s=w4182, f=w4260) -> (s? t:f=w4264:dbl[])
        n2824 = feedback-in #21(w4264) -> ()
        n2825 = Select(t=w4183, s=w4182, f=w4184) -> (s? t:f=w4166:dbl[])
        n2826 = feedback-in #22(w4166) -> ()
        n2827 = local read "Scan lines (y)"() -> (w4151:u64)
        n2828 = local read "N APD Samp/step"() -> (w4167:dbl)
        n2829 = feedback #23(w4209) -> (w4266:dbl[])
        n2830 = Build Array (concatenate)(w4266, w4209) -> (w4257:dbl[])
        n2831 = feedback #24(w4216) -> (w4276:dbl[])
        n2832 = Build Array (concatenate)(w4276, w4216) -> (w4275:dbl[])
        n2833 = feedback #25(w4211) -> (w4268:dbl[])
        n2834 = Build Array (concatenate)(w4268, w4211) -> (w4269:dbl[])
        n2835 = Select(t=w4209, s=w4182, f=w4257) -> (s? t:f=w4213:dbl[])
        n2836 = feedback-in #23(w4213) -> ()
        n2837 = Select(t=w4216, s=w4182, f=w4275) -> (s? t:f=w4215:dbl[])
        n2838 = feedback-in #24(w4215) -> ()
        n2839 = Select(t=w4211, s=w4182, f=w4269) -> (s? t:f=w4214:dbl[])
        n2840 = feedback-in #25(w4214) -> ()
        n2841 = Multiply(x=w4165, y=u64 2) -> (x*y=w4150:u64)
        n2842 = call "integrate 1D array interval - double.vi"("Ave N"=w4167, "Array In"=w4166) -> ("Array Out"=w4178:dbl[])  [unwired: 1 out]
        n2843 = call "integrate 1D array interval - double.vi"("Ave N"=w4167, "Array In"=w4264) -> ("Array Out"=w4263:dbl[])  [unwired: 1 out]
        n2844 = Array Size(array=w4178) -> (size(s)=w4179:i32)
        n2845 = Array Size(array=w4263) -> (size(s)=w4265:i32)
        n2846 = Multiply(x=w4151, y=w4150) -> (x*y=w4181:u64)
        n2847 = Multiply(x=w4151, y=w4150) -> (x*y=w4273:u64)
        n2848 = call-poly <vilib>:"Mean.vi"("X"=w4213) -> ("mean"=w4197:dbl)  [unwired: 1 out]
        n2849 = Subtract(x=w4181, y=w4179) -> (x-y=w4172:u64)
        n2850 = call-poly <vilib>:"Mean.vi"("X"=w4215) -> ("mean"=w4202:dbl)  [unwired: 1 out]
        n2851 = call-poly <vilib>:"Mean.vi"("X"=w4214) -> ("mean"=w4200:dbl)  [unwired: 1 out]
        n2852 = call-poly <vilib>:"Mean.vi"("X"=w4178) -> ("mean"=w4169:dbl)  [unwired: 1 out]
        n2853 = Subtract(x=w4273, y=w4265) -> (x-y=w4207:u64)
        n2854 = call-poly <vilib>:"Mean.vi"("X"=w4263) -> ("mean"=w4204:dbl)  [unwired: 1 out]
        n2855 = Initialize Array(1.0 ("element"), w4172) -> (w4168:dbl[])
        n2856 = Initialize Array(1.0 ("element"), w4207) -> (w4198:dbl[])
        n2857 = Multiply(x=w4168, y=w4169) -> (x*y=w4170:dbl[])
        n2858 = Multiply(x=w4198, y=w4200) -> (x*y=w4201:dbl[])
        n2859 = Multiply(x=w4198, y=w4202) -> (x*y=w4203:dbl[])
        n2860 = Multiply(x=w4198, y=w4197) -> (x*y=w4199:dbl[])
        n2861 = Multiply(x=w4198, y=w4204) -> (x*y=w4205:dbl[])
        n2862 = Build Array (concatenate)(w4213, w4199) -> (w4267:dbl[])
        n2863 = Build Array (concatenate)(w4215, w4203) -> (w4271:dbl[])
        n2864 = Build Array (concatenate)(w4214, w4201) -> (w4270:dbl[])
        n2865 = Build Array (concatenate)(w4178, w4170) -> (w4180:dbl[])
        n2866 = Build Array (concatenate)(w4263, w4205) -> (w4272:dbl[])
        n2867 = Reshape Array(w4267, w4151, w4150) -> (w4233:dbl[][])
        n2868 = Reshape Array(w4180, w4151, w4150) -> (w4176:dbl[][])
